vi "Tela_Set_Coordenadas.vi"() -> (0 "Saída":bool, 1 "Val Saída":string[](array[string]))   [LabVIEW 2012]
panel:
  in  "8":string
  in  "7":string
  in  "6":string
  in  "5":string
  in  "4":string
  in  "3":string
  in  "2":string
  in  "1":string
  in  "Cancel Button":bool
  in  "OK Button":bool
  # "Set New Coordinate to New Object Entry"
  # "RA\nPM"
  # "DEC\nPM"
  # "TRIG\nP.LAX"
  # "HELIO\nVEL"
  # "NAME"
  # "RA"
  # "DEC"
  # "MAG"
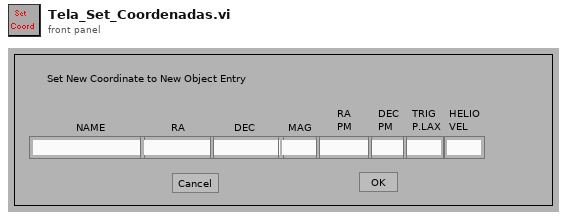
[diagram p1: front panel]
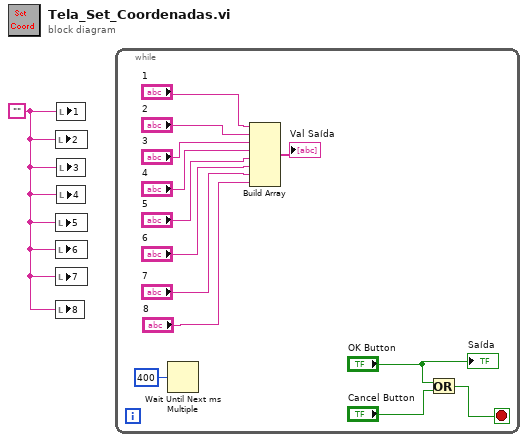
[diagram p0: block diagram]
diagram:
  w1 = ""
  n1 = local write "2"(w1) -> ()
  n2 = local write "5"(w1) -> ()
  n3 = local write "6"(w1) -> ()
  n4 = local write "7"(w1) -> ()
  n5 = local write "8"(w1) -> ()
  n6 = local write "1"(w1) -> ()
  n7 = local write "3"(w1) -> ()
  n8 = local write "4"(w1) -> ()
  n9 = while {
    stop <- w12 stop-if-true
    n10 = Wait Until Next ms Multiple(millisecond multiple=u32 400) -> ()  [unwired: 1 out]
    n11 = Build Array("1", "2", "3", "4", "5", "6", "7", "8") -> (→"Val Saída":string[])
    n12 = Or(x="OK Button", y="Cancel Button") -> (x .or. y?=w12:bool)
    "Saída" <- "OK Button"
  }
